vi "JHOEL_OSORIO_ERICK_TIPAN_AUTOTRONICA_ACTIVIDAD_2.vi"() -> ()   [LabVIEW 2025]
uses:
  <vilib>/express/express arith-compare/Formula/XNode/ExpressFormulaBlockNode.xnode
panel:
  out "CELCIUS":dbl(knob) scale=0.0..100.0
  out "KELVIN":dbl(knob) scale=273.15..373.15
  out "FAHRENHEIT":dbl(knob) scale=32.0..212.0
  out "CELCIUS":dbl
  out "KELVIN":dbl
  out "FAHRENHEIT":dbl
  in  "STOP":bool
  in  "Slide":dbl(slide) scale=0.0..100.0
  out "CALIENTE":bool
  out "FRÍO":bool
  out "CELCIUS":dbl(slide) scale=0.0..100.0
  out "KELVIN":dbl(slide) scale=273.15..373.15
  out "FAHRENHEIT":dbl(slide) scale=32.0..212.0
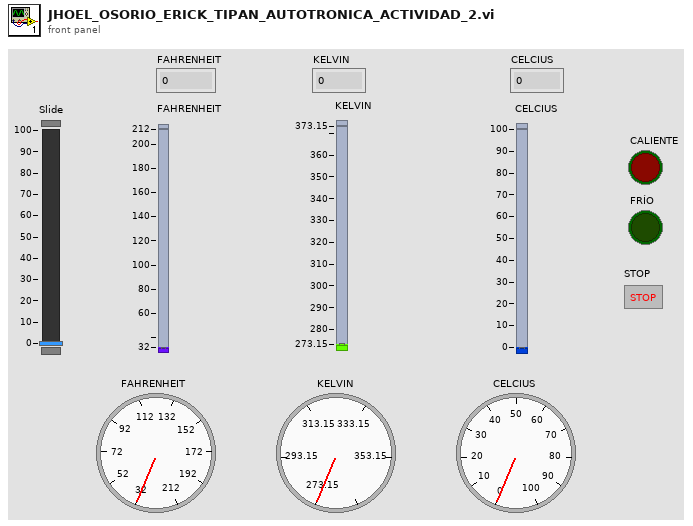
[diagram p1: front panel]
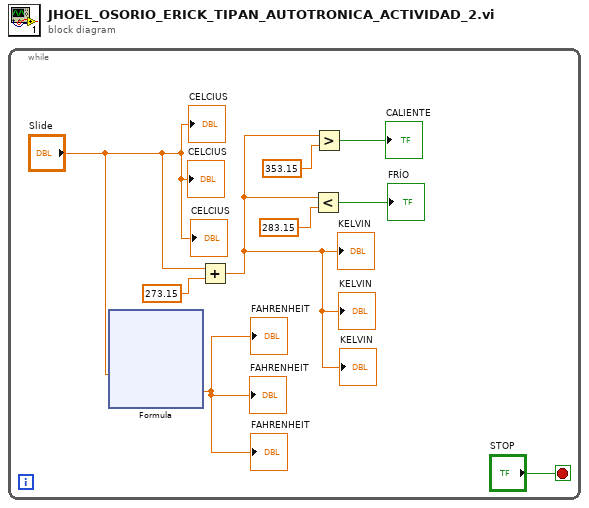
[diagram p0: block diagram]
diagram:
  n1 = while {
    stop <- "STOP" stop-if-true
    n2 = xnode "Formula"("X1"="Slide") -> ("Result"=→"FAHRENHEIT" →"FAHRENHEIT" →"FAHRENHEIT":dbl)  [unwired: 1 in, 1 out]
    n3 = Add(x="Slide", y=273.15) -> (x+y=w2:dbl)
    "KELVIN" <- w2
    "KELVIN" <- w2
    "KELVIN" <- w2
    n4 = Less?(x=w2, y=283.15) -> (x < y?=→"FRÍO":bool)
    n5 = Greater?(x=w2, y=353.15) -> (0:→"CALIENTE":bool)
    "CELCIUS" <- "Slide"
    "CELCIUS" <- "Slide"
    "CELCIUS" <- "Slide"
  }
